vi "ToscaTTL-Main Thread.vi"(2 "IPC":T1) -> (15 "error out":errorcluster)   [LabVIEW 2020]
uses:
  IPC VIs/Tosca-IPC.ctl
  Classes/Parameters/Parameters.lvclass
  Digital Input VIs/Tosca-DI Queue Data.ctl
  Digital Input VIs/Tosca-Input Event.ctl
  Digital Input VIs/Tosca-Input Criterion.ctl
  epl-vi-lib/Utility VIs/Type Defs/Logic State.ctl
  Typedefs/Tosca-Accumulator.ctl
  Typedefs/Tosca-State AODO.ctl
  Typedefs/Tosca-AO Runtime.ctl
  Typedefs/Tosca-DO Runtime.ctl
  epl-vi-lib/Signal Synthesis VIs/4th Generation/Classes/SignalManager/SignalManager.lvclass
  Typedefs/Tosca-Synapse Start Data.ctl
  IPC VIs/Tosca-Message.ctl
  IPC VIs/Tosca-Message Action.ctl
  Typedefs/Tosca-Thread Type.ctl
  Imaging VIs/Tosca-2P-Notifier Data.ctl
  Typedefs/Tosca-MATLAB Queue Data.ctl
  Visual Stim VIs/Tosca-Grating.ctl
  Visual Stim VIs/Tosca-Grating Type.ctl
  Typedefs/Tosca-File IO Notification.ctl
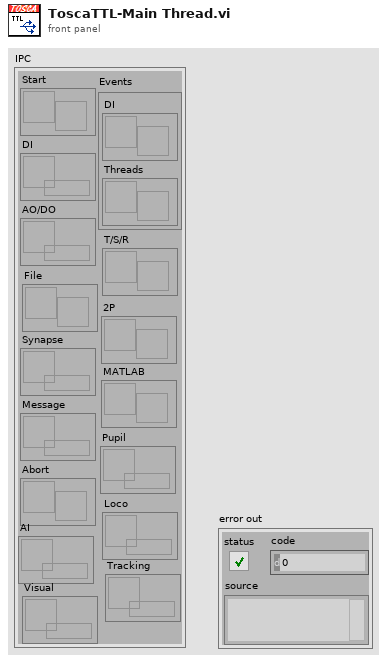
[diagram p1: front panel]
types:
  T1 = typedef "Tosca-IPC.ctl" = cluster{"Start":refnum<notifier>, "DI":refnum<queue>, "AO/DO":refnum<queue>, "Synapse":refnum<queue>, "Message":refnum<queue>, "Abort":refnum<notifier>, "Events":cluster{"DI":refnum<user-event>, "Threads ":refnum<user-event>}, "T/S/R":refnum<notifier>, "2P":refnum<notifier>, "MATLAB":refnum<notifier>, "Pupil":refnum<queue>, "Loco":refnum<queue>, "AI":refnum<queue>, "Tracking":refnum<queue>, "Visual":refnum<queue>, "File":refnum<notifier>}
  T2 = typedef "Tosca-Thread Type.ctl" = enum16{"None", "AODO", "Masker", "ET", "Imaging", "Pupil", "AI", "DI", "Camera", "TTL out", "Loco", "Visual"}
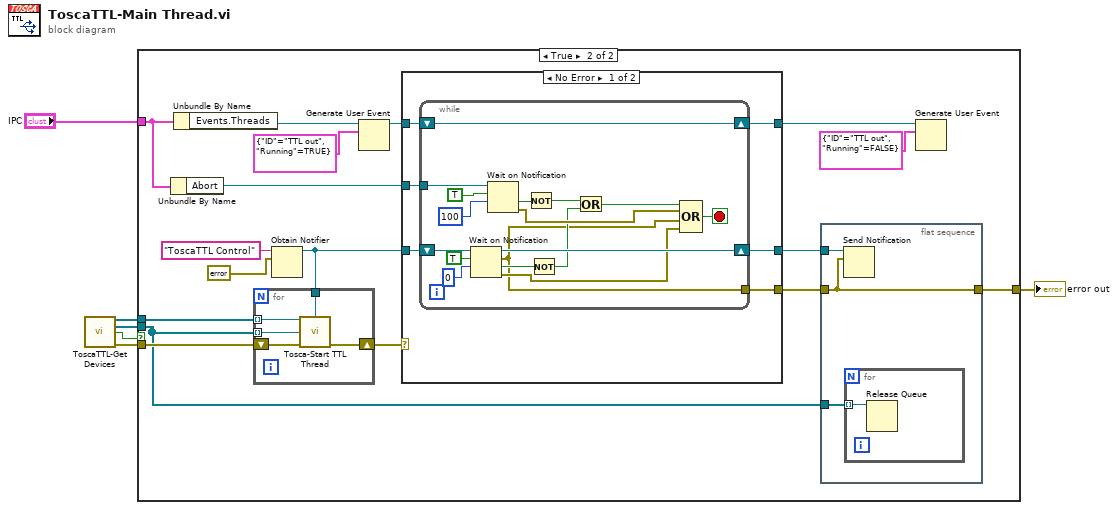
[diagram p0: block diagram]
diagram:
  n1 = call "ToscaTTL-Get Devices.vi"() -> ("Devices"=w4:refnum<class "TTLControlledDevice.lvclass">[], "Queues"=w2:refnum<queue>[], "Any devices?"=w3:bool, "error out"=w1:errorcluster)  [unwired: 12 in]
  n2 = case shown="True" w3 {
    tunnel: "IPC" -> [_ w19]
    tunnel: [w7 w8] -> w5
    tunnel: w4 -> [_ w11]
    tunnel: w2 -> [_ w9]
    tunnel: w1 -> [w7 w10]
    frame False {
    }
    frame True {
      n3 = Unbundle By Name(w19) -> ("Abort"=w18:refnum<notifier>)
      n4 = Unbundle By Name(w19) -> ("Events.Threads"=w24:refnum<user-event>)
      n5 = Obtain Notifier(name (unnamed)="ToscaTTL Control", notification data type=errorcluster {"status"=FALSE, "code"=0, "source"=""} ("error constant")) -> (notifier out=w12:refnum<notifier>)  [unwired: 2 in, 2 out]
      n6 = for {
        tunnel: w11 -> [w59] mode=indexing
        tunnel: w9 -> [w58] mode=indexing
        shift-right: [w57] -> w13
        shift-left: w10 -> [w56]
        tunnel: w12 -> [w55]
        n7 = call "Tosca-Start TTL Thread.vi"("TTLDevice"=w59, "Thread Notifier"=w55, "Control Queue"=w58, "error in (no error)"=w56) -> ("error out"=w57:errorcluster)  [unwired: 11 in]
      }
      n8 = Generate User Event(user event=w24, event data cluster=cluster{"ID":T2, "Running":bool} {"ID"=enum."TTL out", "Running"=TRUE} ("event data")) -> (user event out=w22:refnum<user-event>)  [unwired: 2 in, 1 out]
      n9 = case shown="No Error" w13 {
        selector: w13 -> [_ w52]
        tunnel: w22 -> [w34 w54]
        tunnel: [w33 w54] -> w21
        tunnel: w18 -> [w32 _]
        tunnel: [w31 w53] -> w16
        tunnel: [w30 w52] -> w15
        tunnel: w12 -> [w29 w53]
        frame No Error {
          n10 = while {
            tunnel: w32 -> [w48]
            tunnel: [w36] -> w30
            shift-right: [w51] -> w33
            shift-left: w34 -> [w51]
            shift-right: [w42] -> w31
            shift-left: w29 -> [w43]
            stop <- w46 stop-if-true
            n11 = Wait on Notification(notifier=w43, ignore previous (F)=TRUE, timeout in ms (-1)=0) -> (notifier out=w42:refnum<notifier>, notification=w36:errorcluster, timed out?=w40:bool, error out=w37:errorcluster)  [unwired: 1 in]
            n12 = Wait on Notification(notifier=w48, ignore previous (F)=TRUE, timeout in ms (-1)=100) -> (timed out?=w50:bool, error out=w44:errorcluster)  [unwired: 1 in, 2 out]
            n13 = Not(x=w50) -> (.not. x?=w47:bool)
            n14 = Not(x=w40) -> (.not. x?=w38:bool)
            n15 = Or(x=w47, y=w38) -> (x .or. y?=w39:bool)
            n16 = Compound Arithmetic op=OR(w39, w44, w36, w37) -> (w46:bool)
          }
        }
        frame Error {
        }
      }
      n17 = flat-sequence {
        tunnel: w15 -> [w25]
        tunnel: w16 -> [w27]
        tunnel: w9 -> [w26]
        tunnel: [w25] -> w8
        frame #0 {
          n18 = Send Notification(notification=w25, notifier=w27) -> ()  [unwired: 1 in, 2 out]
          n19 = for {
            tunnel: w26 -> [w28] mode=indexing
            n20 = Release Queue(queue=w28) -> ()  [unwired: 2 in, 3 out]
          }
        }
      }
      n21 = Generate User Event(user event=w21, event data cluster=cluster{"ID":T2, "Running":bool} {"ID"=enum."TTL out", "Running"=FALSE} ("event data")) -> ()  [unwired: 2 in, 2 out]
    }
  }
  "error out" <- w5
